vi "ACC Configuration File Handler.vi"(0 "Operator":T2, 1 "Copy Path":path, 2 "Cfg File Path":path, 7 "Copy Tag":string, 11 "Error In (no error)":errorcluster, 12 "Keys (Empty:All)":T1[](array[typedef]), 13 "Operation":T5) -> (4 "System Configuration Out":T2, 8 "Cancelled":bool, 15 "Error Out":errorcluster)   [LabVIEW 2011]
uses:
  Type Defs/ACTL Access Level Cluster.ctl
  Type Defs/ACTL Operator Cluster.ctl
  Type Defs/ACTL Access Level Enum.ctl
  Configuration Files/Type Defs/CFG File Operation Enum.ctl
  Type Defs/ACTL Configuration Enum.ctl
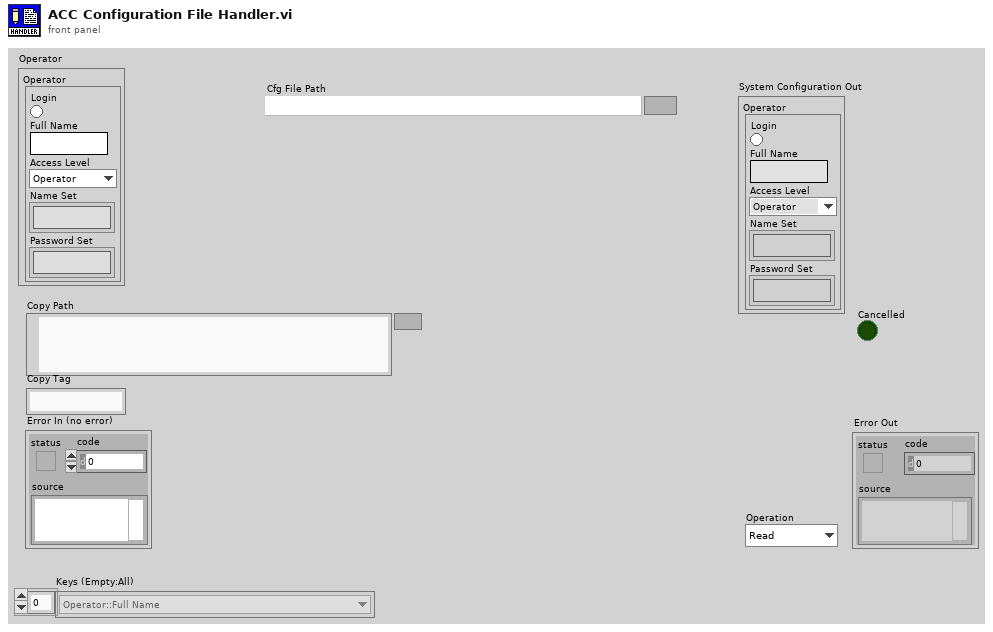
[diagram p1: front panel]
types:
  T1 = typedef "ACTL Configuration Enum.ctl" = enum16{"Operator::Full Name", "Operator::Login", "Operator::Access Level", "Operator::Name Set", "Operator::Password Set"}
  T2 = typedef "ACTL Access Level Cluster.ctl" = cluster{"Operator":T3}
  T3 = typedef "ACTL Operator Cluster.ctl" = cluster{"Full Name":string, "Access Level":T4, "Name Set":string[], "Login":bool, "Password Set":string[]}
  T4 = typedef "ACTL Access Level Enum.ctl" = enum16{"Operator", "Technician", "Engineer", "Programmer"}
  T5 = typedef "CFG File Operation Enum.ctl" = enum16{"Read", "Write", "Copy", "Edit"}
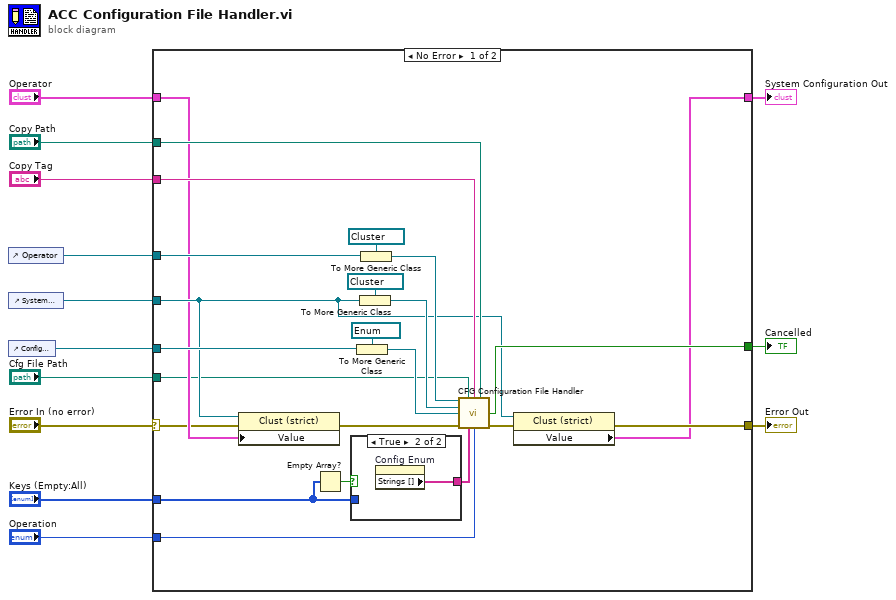
[diagram p0: block diagram]
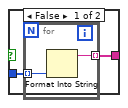
[diagram p2: hidden frame]
diagram:
  n1 = control-ref of="Operator"() -> (w5:refnum<vi>)
  n2 = control-ref of="System Configuration Out"() -> (w4:refnum<vi>)
  n3 = control-ref of="Config Enum"() -> (w3:refnum<vi>)
  n4 = case shown="No Error" "Error In (no error)" {
    selector: "Error In (no error)" -> [w17 w43]
    tunnel: [w16 w43] -> w11
    tunnel: "Copy Path" -> [w35 _]
    tunnel: "Copy Tag" -> [w36 _]
    tunnel: "Operation" -> [w18 _]
    tunnel: [w15 w42] -> w7
    tunnel: "Operator" -> [w19 w42]
    tunnel: w5 -> [w30 _]
    tunnel: w4 -> [w20 _]
    tunnel: w3 -> [w29 _]
    tunnel: "Keys (Empty:All)" -> [w25 _]
    tunnel: [w22 _] -> w2
    tunnel: "Cfg File Path" -> [w14 _]
    frame No Error {
      n5 = property class="Clust (strict)"(reference=w20, error in=w17, "Value"=w19) -> (error out=w21:errorcluster)  [unwired: 1 out]
      n6 = Empty Array?(array=w25) -> (empty?=w24:bool)
      n7 = case shown="True" w24 {
        tunnel: w25 -> [w38 _]
        tunnel: [w37 w41] -> w23
        frame False {
          n8 = for {
            tunnel: w38 -> [w40] mode=indexing
            tunnel: [w39] -> w37 mode=indexing
            n9 = Format Into String(w40) -> (resulting string=w39:string)  [unwired: 3 in, 1 out]
          }
        }
        frame True {
          n10 = property on="Config Enum" class="Enum (strict)"() -> ("Strings []"=w41:string[])  [unwired: 2 in, 2 out]
        }
      }
      n11 = To More Generic Class(target class=refnum<vi> refnum ("Enum Ref"), reference=w29) -> (generic class reference=w26:refnum<vi>)
      n12 = To More Generic Class(target class=refnum<vi> refnum ("Cluster Ref"), reference=w20) -> (generic class reference=w27:refnum<vi>)
      n13 = To More Generic Class(target class=refnum<vi> refnum ("Cluster Ref"), reference=w30) -> (generic class reference=w28:refnum<vi>)
      n14 = call "CFG Configuration File Handler.vi"("Cluster In Ref"=w28, "System Configuration File"=w14, "Copy Tag"=w36, "Copy Path"=w35, "Cluster Out Ref"=w27, "Enum Ref"=w26, "Error In (no error)"=w21, "Keys (Empty:All)"=w23, "Operation"=w18) -> ("Cancelled"=w22:bool, "Error Out"=w34:errorcluster)  [unwired: 1 in, 4 out]
      n15 = property class="Clust (strict)"(reference=w20, error in=w34) -> (error out=w16:errorcluster, "Value"=w15:T2)  [unwired: 1 out]
    }
    frame Error {
    }
  }
  "System Configuration Out" <- w7
  "Error Out" <- w11
  "Cancelled" <- w2
